vi "GenerateAPIEvent_IO.vi"(6 "Timeout (ms)":u32=600000, 7 "Wait (F)":bool, 8 "error in (no error)":errorcluster, 9 "Task ID":string, 10 "API Command Cluster":T1, 11 "IO.lvclass":refnum<class "IO.lvclass">) -> (0 "error out":errorcluster, 3 "IO.lvclass out":refnum<class "IO.lvclass">)   [LabVIEW 2022 SP3, in "IO.lvclass"]
uses:
  IO.lvclass
  Typedefs/API Command Cluster.ctl
  Typedefs/API Command Enum.ctl
  Typedefs/API Event Data.ctl
  Typedefs/API Task State.ctl
  IO.lvclass/IO.ctl
panel:
  out "Return Value":variant
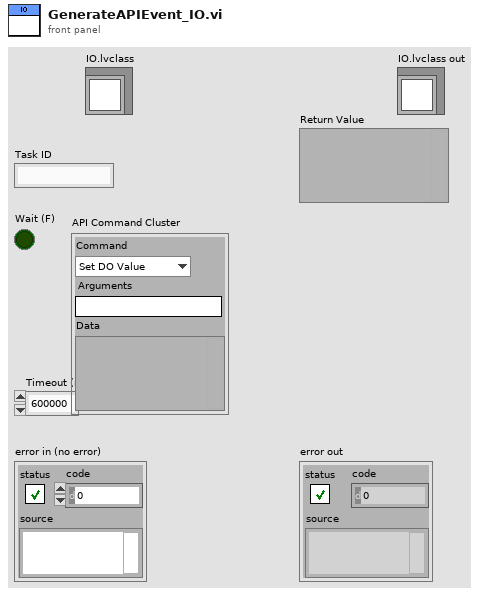
[diagram p1: front panel]
types:
  T1 = typedef "IO.lvclass/API Command Cluster.ctl" = cluster{"Command":T2, "Arguments":string, "Data":variant}
  T2 = typedef "IO.lvclass/API Command Enum.ctl" = enum16{"Set DO Value", "Set AO Value", "Purge PH"}
  T3 = typedef "IO.lvclass/API Task State.ctl" = enum16{"Completed", "Errored", "Pending"}
  T4 = typedef "IO.lvclass/API Event Data.ctl" = cluster{"Task":cluster{"Time Stamp":timestamp, "Timeout (ms)":u32, "Task State":T3, "Task Error":errorcluster, "Task ID":string}, "Command":variant, "Return Value":variant}
  T5 = typedef "IO.lvclass/Private Data.ctl" = cluster{"UserEvents":T6, "All Dependencies":cluster{"Class References":refnum<class>[], "Class Names":string[]}, "Status":T7}
  T6 = typedef "IO.lvclass/UserEvents.ctl" = cluster{"API Incoming Event":refnum<user-event>, "API Executed Event":refnum<user-event>, "API Return Event":refnum<user-event>, "Status Changed Event":refnum<user-event>}
  T7 = typedef "IO.lvclass/Status Cluster.ctl" = cluster{"Device Data":variant, "Ordered ICP1-DO Channels":T8[], "Ordered ICP2-DI Channels":T9[], "Ordered ICP2-DO Channels":T10[], "Ordered ICP1-AI Channels":T11[], "Ordered ICP1-AO Channels":T12[], "Ordered ICP2-AO Channels":T13[]}
  T8 = typedef "IO.lvclass/ICP1-D0 Channel Names.ctl" = enum16{"None", "Meniscus Pressure Reg PWR - R1", "Meniscus Pressure Reg PWR - R2", "Meniscus Pressure Reg PWR - R3", "Meniscus Pressure Reg PWR - R4", "Meniscus Pressure Reg PWR - R5", "Meniscus Pressure Reg PWR - R6", "Clear Stage Alarm", "Servo ON", "Purge Valve Open - R1", "Purge Valve Open - R2", "Purge Valve Open - R3", "Purge Valve Open - R4", "Purge Valve Open - R5", "Purge Valve Open - R6"}
  T9 = typedef "IO.lvclass/ICP2-DI Channel Names.ctl" = enum16{"None", "SW - Ink Valve - R1", "SW - Ink Valve - R2", "SW - Ink Valve - R3", "SW - Ink Valve - R4", "SW - Ink Valve - R5", "SW - Ink Valve - R6", "SW - COVER INPUT SIDE", "SW - COVER OUTPUT SIDE", "SW - Purge - R1", "SW - Purge - R2", "SW - Purge - R3", "SW - Purge - R4", "SW - Purge - R5", "SW - Purge - R6"}
  T10 = typedef "IO.lvclass/ICP2-DO Channel Names.ctl" = enum16{"None", "Meniscus Valve Open - R1", "Meniscus Valve Open - R2", "Meniscus Valve Open - R3", "Meniscus Valve Open - R4", "Meniscus Valve Open - R5", "Meniscus Valve Open - R6", "Ink Flow Valve Open - R1", "Ink Flow Valve Open - R2", "Ink Flow Valve Open - R3", "Ink Flow Valve Open - R4", "Ink Flow Valve Open - R5", "Ink Flow Valve Open - R6", "SW_LED - Ink Valve - R1", "SW_LED - Ink Valve - R2", "SW_LED - Ink Valve - R3", "Recirc Pump On - R1", "Recirc Pump On - R2", "Recirc Pump On - R3", "Recirc Pump On - R4", "Recirc Pump On - R5", "Recirc Pump On - R6", "SW_LED - Ink Valve - R4", "SW_LED - Ink Valve - R5", "SW_LED - Ink Valve - R6"}
  T11 = typedef "IO.lvclass/ICP1-AI Channel Names.ctl" = enum16{"None", "Meniscus Pressure Read - R1", "Meniscus Pressure Read - R2", "Meniscus Pressure Read - R3", "Meniscus Pressure Read - R4", "Meniscus Pressure Read - R5", "Meniscus Pressure Read - R6", "Meniscus Pressure Set - R1", "Meniscus Pressure Set - R2", "Meniscus Pressure Set - R3", "Meniscus Pressure Set - R4", "Meniscus Pressure Set - R5", "Meniscus Pressure Set - R6"}
  T12 = typedef "IO.lvclass/ICP1-AO Channel Names.ctl" = enum16{"None", "Meniscus Pressure Set - R1", "Meniscus Pressure Set - R2", "Meniscus Pressure Set - R3", "Meniscus Pressure Set - R4", "Meniscus Pressure Set - R5", "Meniscus Pressure Set - R6", "Meniscus Vac Pump Speed"}
  T13 = typedef "IO.lvclass/ICP2-AO Channel Names.ctl" = enum16{"None", "Recirc Pump Flow Set - R1", "Recirc Pump Flow Set - R2", "Recirc Pump Flow Set - R3", "Recirc Pump Flow Set - R4", "Recirc Pump Flow Set - R5", "Recirc Pump Flow Set - R6"}
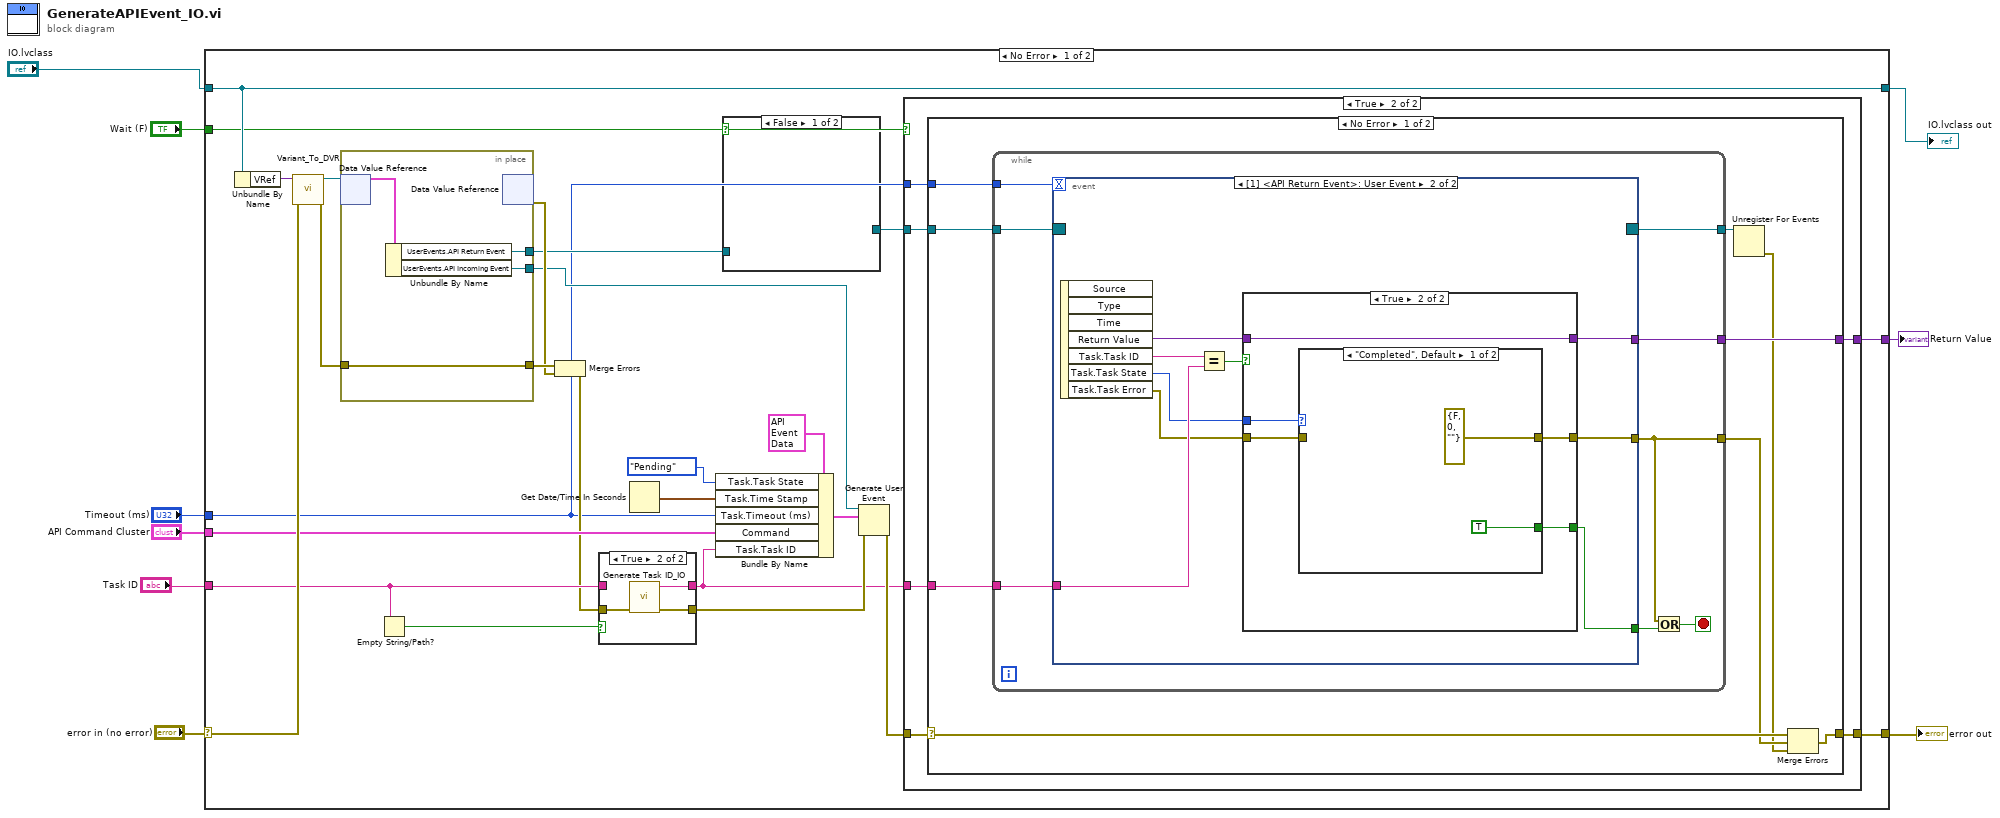
[diagram p0: block diagram]
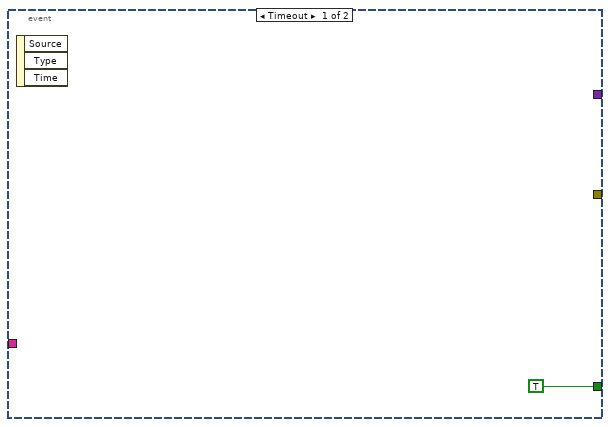
[diagram p4: hidden frame]
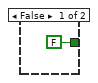
[diagram p5: hidden frame]
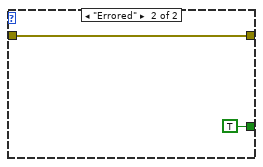
[diagram p6: hidden frame]
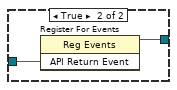
[diagram p8: hidden frame]
diagram:
  n1 = case shown="No Error" "error in (no error)" {
    selector: "error in (no error)" -> [w34 w92]
    tunnel: [w16 w92] -> w8
    tunnel: [w28 w91] -> w2
    tunnel: "IO.lvclass" -> [w28 w91]
    tunnel: "Wait (F)" -> [w21 _]
    tunnel: "Timeout (ms)" -> [w10 _]
    tunnel: "API Command Cluster" -> [w22 _]
    tunnel: [w17 _] -> w4
    tunnel: "Task ID" -> [w14 _]
    frame No Error {
      n2 = Unbundle By Name(w28) -> ("VRef"=w33:variant)
      n3 = call "Variant_To_DVR.vi"("error in (no error)"=w34, "Variant"=w33) -> ("error out"=w31:errorcluster, "DVR"=w32:refnum<data-value>)  [unwired: 8 in]
      n4 = in-place {
        in-place-border: w31 -> [w89]
        in-place-border: [w89] -> w30
        in-place-border: [w88] -> w27
        in-place-border: [w87] -> w26
        n5 = in-place-dvr #1(w32) -> (w90:T5)  [unwired: 1 out]
        n6 = Unbundle By Name(w90) -> ("UserEvents.API Return Event"=w88:refnum<user-event>, "UserEvents.API Incoming Event"=w87:refnum<user-event>)
        n7 = in-place-dvr #1() -> (w29:errorcluster)  [unwired: 1 in, 1 out]
      }
      n8 = Empty String/Path?(string/path=w14) -> (empty?=w15:bool)
      n9 = Merge Errors(w30, w29) -> (w13:errorcluster)
      n10 = case shown="True" w15 {
        tunnel: [w36 w39] -> w11
        tunnel: w14 -> [w36 _]
        tunnel: w13 -> [w35 w38]
        tunnel: [w35 w37] -> w12
        frame False {
        }
        frame True {
          n11 = call "Generate Task ID_IO.vi"("error in (no error)"=w38) -> ("error out"=w37:errorcluster, "Task ID"=w39:string)  [unwired: 9 in]
        }
      }
      n12 = Get Date/Time In Seconds() -> (seconds since 1Jan1904=w24:timestamp)
      n13 = Bundle By Name(cluster=T4 {"Task"={"Time Stamp"=timestamp(0 s since 1904-01-01), "Timeout (ms)"=0, "Task State"=enum."Completed", "Task Error"={"status"=FALSE, "code"=0, "source"=""}, "Task ID"=""}, "Command"=variant, "Return Value"=variant} ("event data"), "Task.Task State"=API_Task_State."Pending", "Task.Time Stamp"=w24, "Task.Timeout (ms)"=w10, "Command"=w22, "Task.Task ID"=w11) -> (w23:T4)
      n14 = case shown="False" w21 {
        tunnel: w27 -> [_ w86]
        tunnel: [_ w85] -> w19
        frame False {
        }
        frame True {
          n15 = register-events(w86) -> (reference out=w85:refnum<event-registration>)  [unwired: 2 in, 1 out]
        }
      }
      n16 = Generate User Event(user event=w26, event data cluster=w23, error in=w12) -> (error out=w20:errorcluster)  [unwired: 1 in, 1 out]
      n17 = case shown="True" w21 {
        tunnel: w20 -> [w40 w46]
        tunnel: w10 -> [_ w45]
        tunnel: w19 -> [_ w44]
        tunnel: [_ w43] -> w17
        tunnel: [w40 w42] -> w16
        tunnel: w11 -> [_ w41]
        frame False {
        }
        frame True {
          n18 = case shown="No Error" w46 {
            selector: w46 -> [w51 w84]
            tunnel: w45 -> [w55 _]
            tunnel: w44 -> [w54 _]
            tunnel: [w53 _] -> w43
            tunnel: [w48 w84] -> w42
            tunnel: w41 -> [w47 _]
            frame No Error {
              n19 = while {
                tunnel: w55 -> [w63]
                tunnel: w54 -> [w62]
                tunnel: [w61] -> w53
                tunnel: [w58] -> w52
                tunnel: [w57] -> w50
                tunnel: w47 -> [w56]
                stop <- w59 stop-if-true
                n20 = event shown="[1] <API Return Event>: User Event" {
                  selector: w62 -> [_ _]
                  dyn-events: [_ _] -> w58
                  timeout: w63 -> [_ _]
                  tunnel: [_ w70] -> w61
                  tunnel: [_ w66] -> w57
                  tunnel: [TRUE w65] -> w60
                  tunnel: w56 -> [_ w72]
                  event Timeout {
                    n21 = event-data() -> ()  [unwired: 1 in, 3 out]
                  }
                  event User Event {
                    n22 = event-data() -> ("Return Value"=w71:variant, "Task.Task ID"=w73:string, "Task.Task State"=w68:T3, "Task.Task Error"=w67:errorcluster)  [unwired: 1 in, 3 out]
                    n23 = Equal?(x=w73, y=w72) -> (x = y?=w69:bool)
                    n24 = case shown="True" w69 {
                      tunnel: w68 -> [_ w79]
                      tunnel: w67 -> [_ w78]
                      tunnel: [_ w77] -> w70
                      tunnel: w71 -> [_ w77]
                      tunnel: [_ w76] -> w66
                      tunnel: [FALSE w75] -> w65
                      frame False {
                      }
                      frame True {
                        n25 = case shown="\"Completed\", Default" w79 {
                          tunnel: w78 -> [_ w83]
                          tunnel: [errorcluster {"status"=FALSE, "code"=0, "source"=""} ("Task Error") w83] -> w76
                          tunnel: [TRUE TRUE] -> w75
                          frame "Completed", Default {
                          }
                          frame "Errored" {
                          }
                        }
                      }
                    }
                  }
                }
                n26 = Or(x=w57, y=w60) -> (x .or. y?=w59:bool)
              }
              n27 = Unregister For Events(event registration refnum=w52) -> (error out=w49:errorcluster)  [unwired: 1 in]
              n28 = Merge Errors(w51, w50, w49) -> (w48:errorcluster)
            }
            frame Error {
            }
          }
        }
      }
    }
    frame Error {
    }
  }
  "error out" <- w8
  "Return Value" <- w4
  "IO.lvclass out" <- w2
